vi "ChannelSelectionScreen.vi"(7 "Generate?":bool, 8 "error in":errorcluster, 10 "Frame Configuration":T2 {"CRCConfiguration"."FinalXorValue" format="%0x"; "CRCConfiguration"."InitialCRC" format="%0x"; "CRCConfiguration"."Polynomial" format="%0x"; "CRC"."Data Type" items=["Signed", "Unsigned", "IEEE Float"]; "Rolling Counter"."Data Type" items=["Signed", "Unsigned", "IEEE Float"]; "Input Channels"."Data Type" items=["Signed", "Unsigned", "IEEE Float"]}, 11 "Parent Ref":T5=18446744073709551615 format="%.0x") -> (0 "error out":errorcluster, 1 "Cancelled?":bool, 2 "Frame Configuration out":T2 {"CRCConfiguration"."FinalXorValue" format="%0x"; "CRCConfiguration"."InitialCRC" format="%0x"; "CRCConfiguration"."Polynomial" format="%0x"; "CRC"."Data Type" items=["Signed", "Unsigned", "IEEE Float"]; "Rolling Counter"."Data Type" items=["Signed", "Unsigned", "IEEE Float"]; "Input Channels"."Data Type" items=["Signed", "Unsigned", "IEEE Float"]}, 3 "Parent Ref Out":T5=18446744073709551615 format="%.0x")   [LabVIEW 2021, in "LIN Frame Protection Addon System Explorer.lvlib"]
uses:
  LIN Frame Protection Addon System Explorer.lvlib
  NationalInstruments.VeriStand.SystemStorageUI
  <vilib>/NI VeriStand/Custom Device API/Custom Device Item Ref.ctl
  Shared/Types/FrameConfiguration.ctl
  Shared/Types/InputChannelConfiguration.ctl
  Shared/Types/Protection Type.ctl
  Shared/Types/CRCConfiguration.ctl
  <vilib>/NI VeriStand/Custom Device API/Custom Device API.lvlib
  <vilib>/NI VeriStand/Custom Device Tools/Custom Device Utility Library/Custom Device Utility Library.lvlib
  Shared/LIN Frame Protection Addon Shared.lvlib
panel:
  in  "Reflected":bool
  in  "Final Xor Value":u32 format="%.0x"
  in  "Inital CRC":u32 format="%.0x"
  in  "Polynomial":u32 format="%0x"
  in  "Protection Type":T1
  in  "Protection":refnum<k24>(container)
  in  "Max Count":dbl=4.0
  in  "Rolling Counter":refnum<k24>(container)
  in  "Cancel":bool
  in  "OK":bool
  in  "Protection Data":refnum<k24>(container)
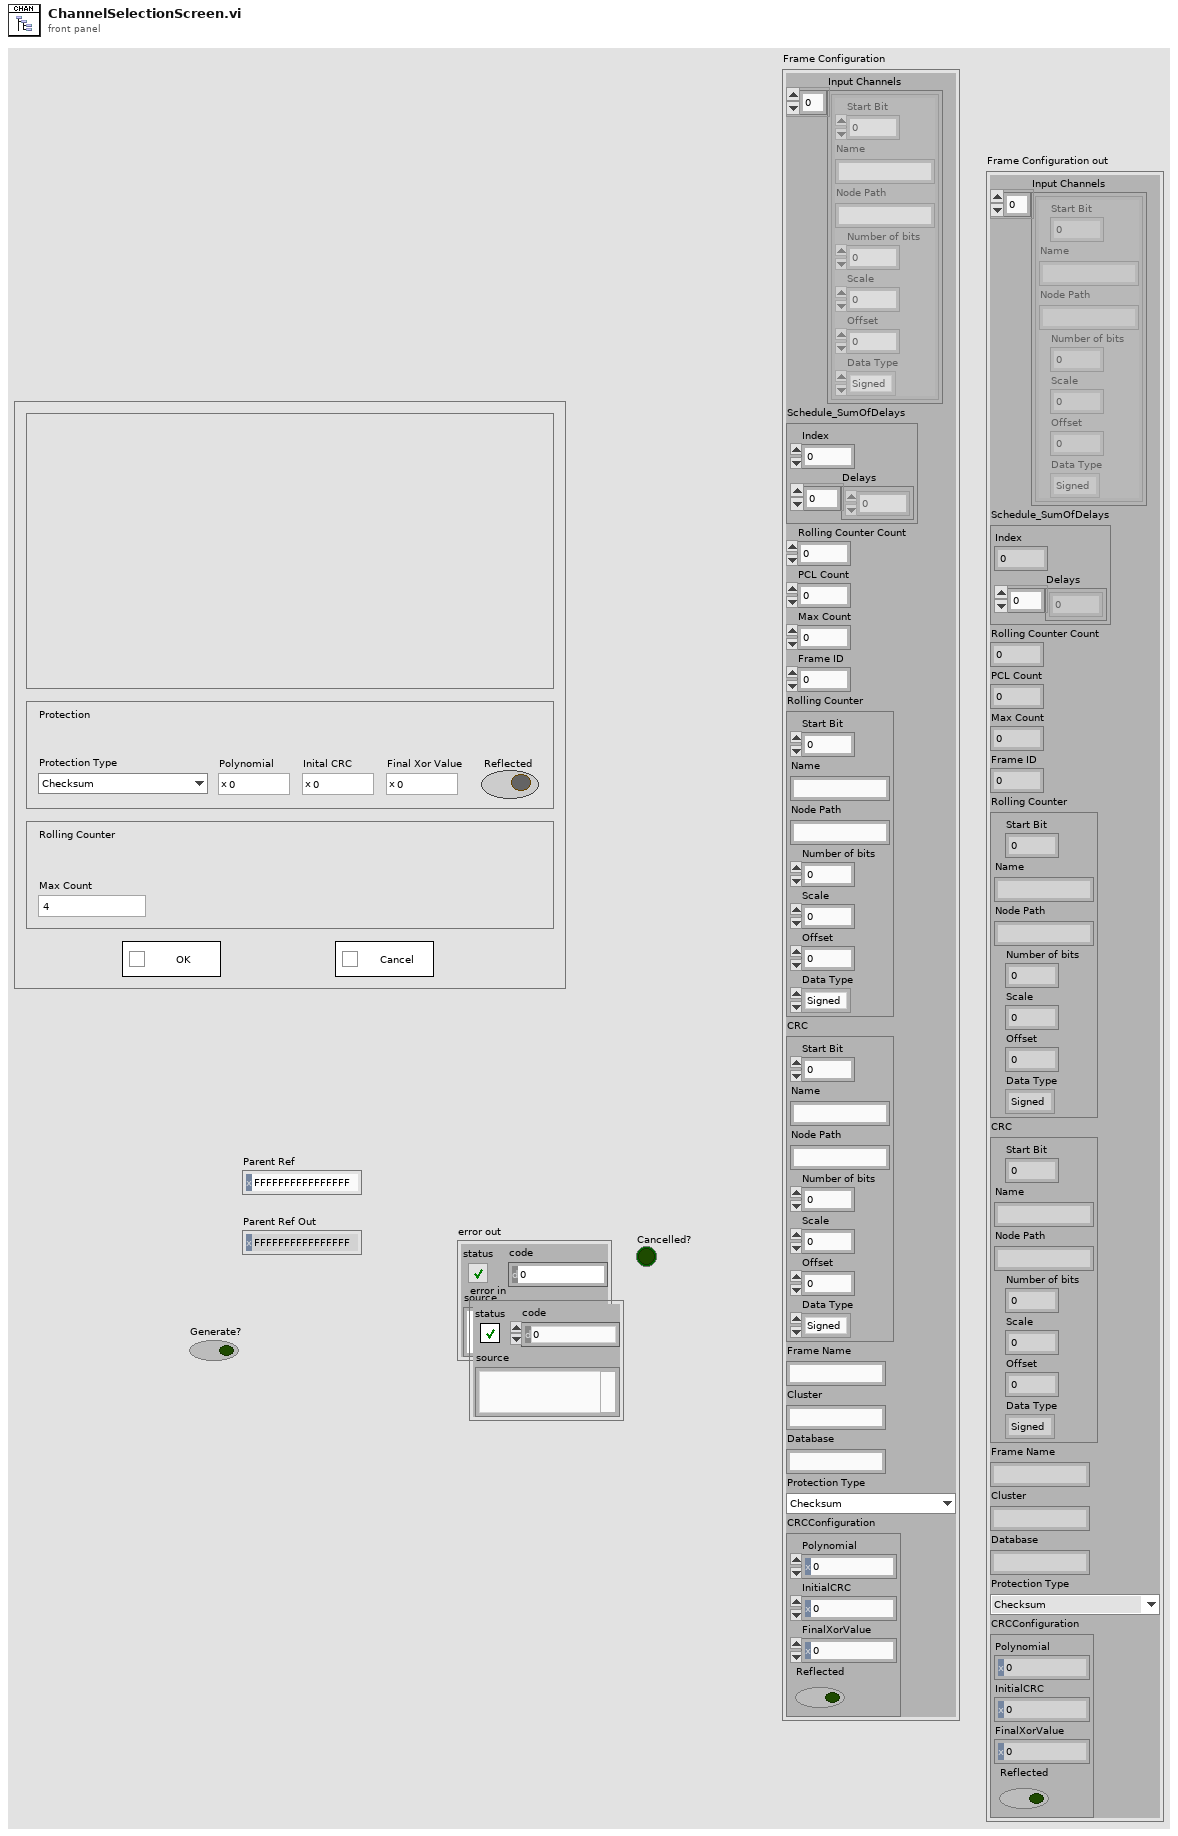
[diagram p1: front panel]
types:
  T1 = typedef "LIN Frame Protection Addon Shared.lvlib/Protection Type.ctl" = enum16{"Checksum", "CRC-8", "CRC-16", "CRC-32", "None (Counter Only)"}
  T2 = typedef "LIN Frame Protection Addon Shared.lvlib/FrameConfiguration.ctl" = cluster{"Input Channels":T3[], "Schedule_SumOfDelays":cluster{"Index":i32, "Delays":dbl[]}, "Rolling Counter Count":dbl, "PCL Count":u64, "Max Count":dbl, "Frame ID":u32, "Rolling Counter":T3, "CRC":T3, "Frame Name":string, "Cluster":string, "Database":string, "Protection Type":T1, "CRCConfiguration":T4}
  T3 = typedef "LIN Frame Protection Addon Shared.lvlib/InputChannelConfiguration.ctl" = cluster{"Start Bit":i32, "Name":string, "Node Path":string, "Number of bits":i32, "Scale":dbl, "Offset":dbl, "Data Type":u32}
  T4 = typedef "LIN Frame Protection Addon Shared.lvlib/CRCConfiguration.ctl" = cluster{"Polynomial":u64, "InitialCRC":u64, "FinalXorValue":u64, "Reflected":bool}
  T5 = typedef "Custom Device API.lvlib/Custom Device Item Ref.ctl" = u64
  T6 = typedef "Custom Device API.lvlib/Custom Device Pointer.ctl" = refnum<k24>
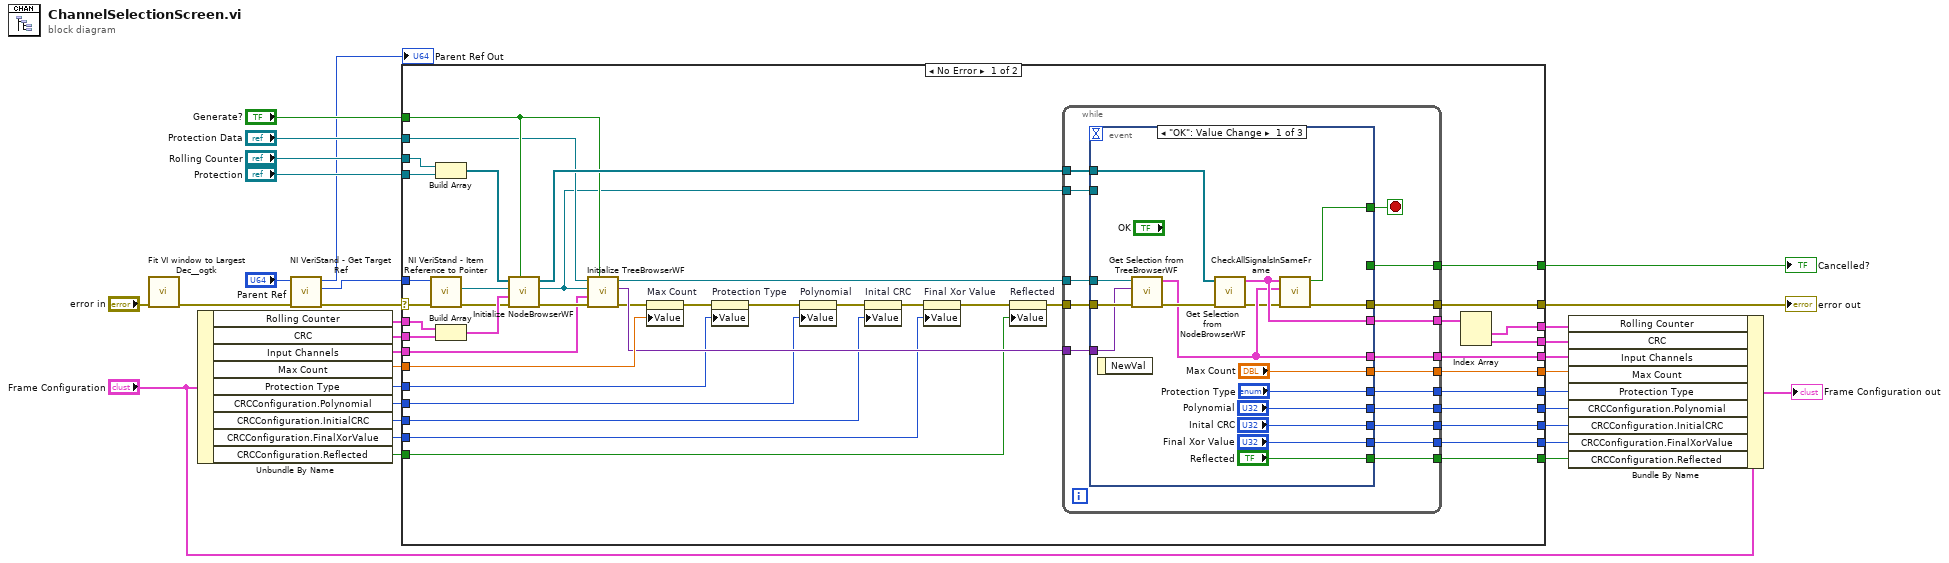
[diagram p0: block diagram]
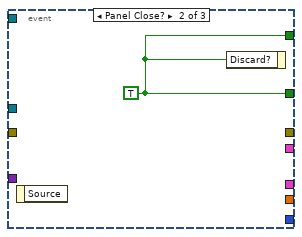
[diagram p2: hidden frame]
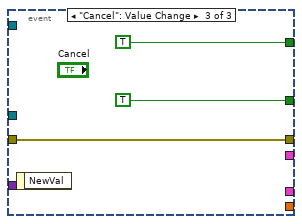
[diagram p3: hidden frame]
diagram:
  n1 = call <userlib>:"Fit VI window to Largest Dec__ogtk.vi"("error in (no error)"="error in") -> ("error out"=w6:errorcluster)  [unwired: 5 in, 1 out]
  n2 = Unbundle By Name("Frame Configuration") -> ("Rolling Counter"=w21:T3, "CRC"=w20:T3, "Input Channels"=w27:T3[], "Max Count"=w16:dbl, "Protection Type"=w5:T1, "CRCConfiguration.Polynomial"=w4:u64, "CRCConfiguration.InitialCRC"=w3:u64, "CRCConfiguration.FinalXorValue"=w2:u64, "CRCConfiguration.Reflected"=w1:bool)
  n3 = call <vilib>:"NI VeriStand - Get Target Ref.vi"("error in"=w6, "Item Ref in"="Parent Ref") -> ("error out"=w29:errorcluster, "Target Ref"=w13:T5, "Item Ref out"=→"Parent Ref Out":T5)  [unwired: 6 in, 1 out]
  n4 = case shown="No Error" w29 {
    selector: w29 -> [w74 w112]
    tunnel: "Protection Data" -> [w55 _]
    tunnel: w13 -> [w75 _]
    tunnel: [w73 _] -> w31
    tunnel: [w49 w112] -> w30
    tunnel: [w72 _] -> w26
    tunnel: w27 -> [w63 _]
    tunnel: "Rolling Counter" -> [w70 _]
    tunnel: "Protection" -> [w71 _]
    tunnel: w21 -> [w69 _]
    tunnel: w20 -> [w68 _]
    tunnel: [w60 _] -> w19
    tunnel: [w59 _] -> w18
    tunnel: [w58 _] -> w17
    tunnel: w16 -> [w57 _]
    tunnel: "Generate?" -> [w56 _]
    tunnel: [w48 _] -> w12
    tunnel: [w47 _] -> w11
    tunnel: [w46 _] -> w10
    tunnel: [w45 _] -> w9
    tunnel: [w44 _] -> w8
    tunnel: w5 -> [w37 _]
    tunnel: w4 -> [w36 _]
    tunnel: w3 -> [w35 _]
    tunnel: w2 -> [w34 _]
    tunnel: w1 -> [w33 _]
    frame No Error {
      n5 = call <vilib>:"NI VeriStand - Item Reference to Pointer.vi"("error in (no error)"=w74, "Item Ref in"=w75) -> ("error out"=w66:errorcluster, "Node Pointer"=w54:T6)  [unwired: 6 in, 2 out]
      n6 = Build Array(w70, w71) -> (w64:refnum<k24>[])
      n7 = Build Array(w69, w68) -> (w67:T3[])
      n8 = call "Initialize NodeBrowserWF.vi"("Generate?"=w56, "error in (no error)"=w66, "Output Channels"=w67, "Node Pointer"=w54, "NodeBrowserRefs"=w64) -> ("error out"=w65:errorcluster, "Node Pointer"=w52:T6, "NodeBrowserRefs"=w62:refnum<k24>[])  [unwired: 4 in]
      n9 = call "Initialize TreeBrowserWF.vi"("Generate?"=w56, "error in (no error)"=w65, "Input Channels"=w63, "Node Pointer"=w52, "TreeBrowserRef"=w55) -> ("error out"=w50:errorcluster, "Channels"=w53:variant, "TreeBrowserRef 2"=w51:refnum<k24>)  [unwired: 4 in]
      n10 = property on="Max Count" class="DigNum (strict)"(error in=w50, "Value"=w57) -> (error out=w43:errorcluster)  [unwired: 1 in, 1 out]
      n11 = property on="Protection Type" class="Enum (strict)"(error in=w43, "Value"=w37) -> (error out=w42:errorcluster)  [unwired: 1 in, 1 out]
      n12 = property on="Polynomial" class="DigNum (strict)"(error in=w42, "Value"=w36) -> (error out=w38:errorcluster)  [unwired: 1 in, 1 out]
      n13 = property on="Inital CRC" class="DigNum (strict)"(error in=w38, "Value"=w35) -> (error out=w39:errorcluster)  [unwired: 1 in, 1 out]
      n14 = property on="Final Xor Value" class="DigNum (strict)"(error in=w39, "Value"=w34) -> (error out=w41:errorcluster)  [unwired: 1 in, 1 out]
      n15 = property on="Reflected" class="Bool (strict)"(error in=w41, "Value"=w33) -> (error out=w40:errorcluster)  [unwired: 1 in, 1 out]
      n16 = while {
        tunnel: w40 -> [w91]
        tunnel: w51 -> [w90]
        tunnel: [w88] -> w73
        tunnel: [w87] -> w49
        tunnel: [w86] -> w72
        tunnel: w53 -> [w85]
        tunnel: w62 -> [w84]
        tunnel: [w83] -> w61
        tunnel: [w82] -> w58
        tunnel: w52 -> [w81]
        tunnel: [w80] -> w48
        tunnel: [w79] -> w47
        tunnel: [w78] -> w46
        tunnel: [w77] -> w45
        tunnel: [w76] -> w44
        stop <- w89 stop-if-true
        n17 = event shown="[0] \"OK\": Value Change" {
          selector: _ -> [_ _ _]
          dyn-events: _ -> [_ _ _]
          timeout: _ -> [_ _ _]
          tunnel: w91 -> [w107 _ w111]
          tunnel: w90 -> [w106 _ _]
          tunnel: [w99 _ w111] -> w87
          tunnel: [w98 w108 TRUE] -> w89
          tunnel: [_ w108 TRUE] -> w88
          tunnel: [w101 _ _] -> w86
          tunnel: w85 -> [w105 _ _]
          tunnel: w84 -> [w104 _ _]
          tunnel: [w102 _ _] -> w83
          tunnel: ["Max Count" _ _] -> w82
          tunnel: w81 -> [_ _ _]
          tunnel: ["Protection Type" _ _] -> w80
          tunnel: ["Polynomial" _ _] -> w79
          tunnel: ["Inital CRC" _ _] -> w78
          tunnel: ["Final Xor Value" _ _] -> w77
          tunnel: ["Reflected" _ _] -> w76
          event "OK": Value Change {
            n18 = event-data() -> ()  [unwired: 1 in, 1 out]
            n19 = call "Get Selection from TreeBrowserWF.vi"("error in (no error)"=w107, "Input Channels"=w105, ".NET Refnum in"=w106) -> ("error out"=w103:errorcluster, "Input Channel Selections"=w101:T3[])  [unwired: 7 in]
            n20 = call "Get Selection from NodeBrowserWF.vi"("error in (no error)"=w103, "NodeBrowserRefs"=w104) -> ("error out"=w100:errorcluster, "Array"=w102:T3[])  [unwired: 8 in]
            n21 = call "CheckAllSignalsInSameFrame.vi"("error in"=w100, "Input Channel Selections"=w101, "Rolling Counter and CRC"=w102) -> ("error out"=w99:errorcluster, "Pass?"=w98:bool)  [unwired: 7 in]
          }
          event Panel Close? {
            w108 = TRUE
            n22 = event-data() -> ()  [unwired: 1 in, 1 out]
            n23 = event-data("Discard?"=w108) -> ()  [unwired: 1 in, 1 out]
          }
          event "Cancel": Value Change {
            n24 = event-data() -> ()  [unwired: 1 in, 1 out]
          }
        }
      }
      n25 = Index Array(array=w61) -> (element #1=w59:T3, element #2=w60:T3)  [unwired: 2 in]
    }
    frame Error {
    }
  }
  "Cancelled?" <- w31
  "error out" <- w30
  n26 = Bundle By Name(cluster="Frame Configuration", "Rolling Counter"=w18, "CRC"=w19, "Input Channels"=w26, "Max Count"=w17, "Protection Type"=w12, "CRCConfiguration.Polynomial"=w11, "CRCConfiguration.InitialCRC"=w10, "CRCConfiguration.FinalXorValue"=w9, "CRCConfiguration.Reflected"=w8) -> (→"Frame Configuration out":T2)
